vi "Hough Line Transform.vi"() -> ()   [LabVIEW 2018]
doc: "Hough Line Transform: This example is an example of Hough Line Transform, which considers each pixel in an image to be possibly on certain lines. The goal of this example is to find parameters in the Hough space that can explain the straight lines in the image."
uses:
  vi.lib/VIRobotics/opencv_yiku/ctls/ColorConversionCodes.ctl
  vi.lib/VIRobotics/opencv_yiku/Mat/Mat_8U/Mat_8U.lvclass
  D:/Program Files/Company/National Instruments/LabVIEW 2018(64bit)/vi.lib/addons/VIRobotics/opencv_yiku/Mat/Mat/Mat.lvclass
  vi.lib/VIRobotics/opencv_yiku/Mat/Create_Mat_8U.vi
  vi.lib/VIRobotics/opencv_yiku/opencv_yiku.lvlib
panel:
  out "lines":cluster{"distance":sgl, "theta":sgl}[](array[cluster])
  in  "parameters":T1={"rho"=1.0, "theta"=0.017453292519943295, "threshold"=200, "srn"=20.0, "stn"=10.0, "min_theta"=0.0, "max_theta"=3.141592653589793}
  out "lines":picture
  out "canny":picture
  out "picture":picture
  # "Overview: Demonstrates how to detect lines in an image.\nRequirements: Windows.\nInstructions: \n1.Run the VI"
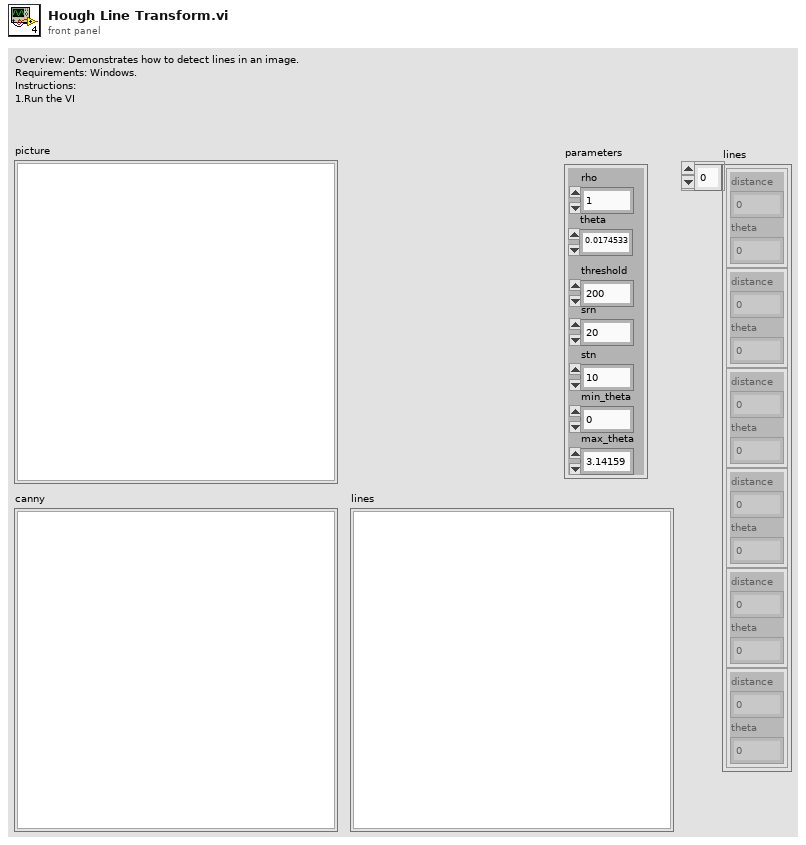
[diagram p1: front panel]
types:
  T1 = cluster{"rho":dbl, "theta":dbl, "threshold":i32, "srn":dbl, "stn":dbl, "min_theta":dbl, "max_theta":dbl}
  T2 = typedef "opencv_yiku.lvlib/ColorConversionCodes.ctl" = enum32{"COLOR_BGR2BGRA", "COLOR_BGRA2BGR", "COLOR_BGR2RGBA", "COLOR_RGBA2BGR", "COLOR_BGR2RGB", "COLOR_BGRA2RGBA", "COLOR_BGR2GRAY", "COLOR_RGB2GRAY", "COLOR_GRAY2BGR", "COLOR_GRAY2BGRA", "COLOR_BGRA2GRAY", "COLOR_RGBA2GRAY", "COLOR_BGR2BGR565", "COLOR_RGB2BGR565", "COLOR_BGR5652BGR", "COLOR_BGR5652RGB", "COLOR_BGRA2BGR565", "COLOR_RGBA2BGR565", "COLOR_BGR5652BGRA", "COLOR_BGR5652RGBA", "COLOR_GRAY2BGR565", "COLOR_BGR5652GRAY", "COLOR_BGR2BGR555", "COLOR_RGB2BGR555", "COLOR_BGR5552BGR", "COLOR_BGR5552RGB", "COLOR_BGRA2BGR555", "COLOR_RGBA2BGR555", "COLOR_BGR5552BGRA", "COLOR_BGR5552RGBA", "COLOR_GRAY2BGR555", "COLOR_BGR5552GRAY", "COLOR_BGR2XYZ", "COLOR_RGB2XYZ", "COLOR_XYZ2BGR", "COLOR_XYZ2RGB", "COLOR_BGR2YCrCb", "COLOR_RGB2YCrCb", "COLOR_YCrCb2BGR", "COLOR_YCrCb2RGB", "COLOR_BGR2HSV", "COLOR_RGB2HSV", "42", "43", "COLOR_BGR2Lab", "COLOR_RGB2Lab"}
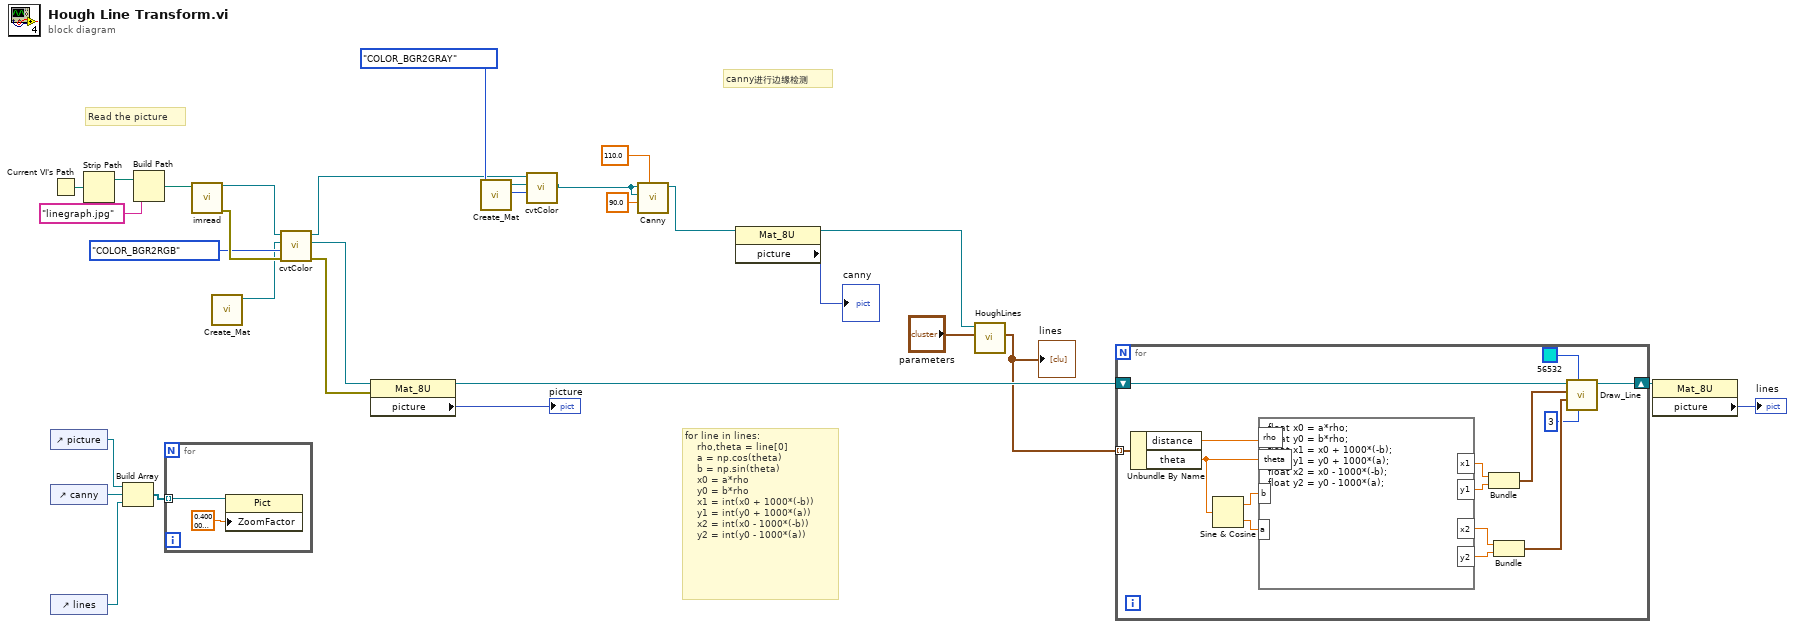
[diagram p0: block diagram]
diagram:
  # "Read the picture"
  # "for line in lines:\n    rho,theta = line[0]\n    a = np.cos(theta)\n    b = np.sin(theta)\n    x0 = a*rho\n    y0 = b*rho\n    x1 = int(x0 + 1000*(-b))\n    y1 = int(y0 + 1000*(a))\n    x2 = int(x0 - 1000*(-b))\n    y2 = int(y0 - 1000*(a))"
  # "canny进行边缘检测"
  n1 = Current VI's Path() -> (path=w27:path)
  n2 = control-ref of="picture"() -> (w17:refnum<vi>)
  n3 = control-ref of="canny"() -> (w16:refnum<vi>)
  n4 = control-ref of="lines"() -> (w4:refnum<vi>)
  n5 = Strip Path(path=w27) -> (stripped path=w29:path)  [unwired: 1 out]
  n6 = Build Array(w17, w16, w4) -> (w15:refnum<vi>[])
  n7 = Build Path(base path=w29, name or relative path="linegraph.jpg") -> (appended path=w26:path)
  n8 = for {
    tunnel: w15 -> [w31] mode=indexing
    n9 = property class="Pict"(reference=w31, "ZoomFactor"=sgl 0.4 ("Zoom Factor")) -> ()  [unwired: 1 in, 2 out]
  }
  n10 = call "imread.vi"("path"=w26) -> ("error out"=w21:errorcluster, "Mat out"=w22:refnum<class "Mat_8U.lvclass">)  [unwired: 9 in]
  n11 = call-poly "Create_Mat.vi"() -> ("Mat_8U_out"=w12:refnum<class "Mat_8U.lvclass">)  [unwired: 10 in, 1 out]
  n12 = call "cvtColor.vi"("error in (no error)"=w21, "dstCn"=ColorConversionCodes."COLOR_BGR2RGB", "dst"=w12, "src"=w22) -> ("error out"=w20:errorcluster, "dst out"=w11:refnum<class "Mat_8U.lvclass">, "src out"=w10:refnum<class "Mat_8U.lvclass">)  [unwired: 5 in]
  n13 = property class="Mat_8U"(reference=w11, error in=w20) -> (reference out=w9:refnum<class "Mat_8U.lvclass">, "picture"=→"picture":picture)  [unwired: 1 out]
  n14 = call-poly "Create_Mat.vi"() -> ("Mat_8U_out"=w23:refnum<class "Mat_8U.lvclass">)  [unwired: 10 in, 1 out]
  n15 = call "cvtColor.vi"("dstCn"=ColorConversionCodes."COLOR_BGR2GRAY", "dst"=w23, "src"=w10) -> ("dst out"=w3:refnum<class "Mat_8U.lvclass">)  [unwired: 6 in, 2 out]
  n16 = call "Canny.vi"("threshold2"=110.0, "threshold1"=90.0, "dst in"=w3, "Mat in"=w3) -> ("dst out"=w6:refnum<class "Mat_8U.lvclass">)  [unwired: 6 in, 1 out]
  n17 = property class="Mat_8U"(reference=w6) -> (reference out=w5:refnum<class "Mat_8U.lvclass">, "picture"=→"canny":picture)  [unwired: 1 in, 1 out]
  n18 = call "HoughLines.vi"("parameters"="parameters", "Mat in"=w5) -> ("lines"=w1:cluster{"distance":sgl, "theta":sgl}[])  [unwired: 7 in, 2 out]
  "lines" <- w1
  n19 = for {
    shift-right: [w40] -> w14
    shift-left: w9 -> [w41]
    tunnel: w1 -> [w46] mode=indexing
    n20 = Unbundle By Name(w46) -> ("distance"=w45:sgl, "theta"=w43:sgl)
    n21 = Sine & Cosine(0:w43) -> (1:w42:sgl, 2:w44:sgl)
    n22 = formula code="float x0 = a*rho;\nfloat y0 = b*rho;\nfloat x1 = x0 + 1000*(-b);\nfloat y1 = y0 + 1000*(a);\nfloat x2 = x0 - 1000*(-b);\nfloat y2 = y0 - 1000*(a);"("theta"=w43, "rho"=w45, "b"=w42, "a"=w44) -> ("x1"=w39:dbl, "y1"=w38:dbl, "x2"=w36:dbl, "y2"=w35:dbl)
    n23 = Bundle(w39, w38) -> (w37:cluster{dbl, dbl})  [unwired: 1 in]
    n24 = Bundle(w36, w35) -> (w34:cluster{dbl, dbl})  [unwired: 1 in]
    n25 = call "Draw_Line.vi"("thickness"=3, "color"=u32 56532, "pt2"=w34, "pt1"=w37, "Mat"=w41) -> ("Mat out"=w40:refnum<class "Mat_8U.lvclass">)  [unwired: 5 in, 1 out]
  }
  n26 = property class="Mat_8U"(reference=w14) -> ("picture"=→"lines":picture)  [unwired: 1 in, 2 out]
